vi "Average_IBP_curves_baseline.vi"(0 "I in":dbl[](array[numeric]), 1 "Averaged P(B) In":dbl[][](array[numeric]), 2 "Counter":i8, 3 "B0":dbl, 5 "Averaged I(B) In":dbl[][](array[numeric]), 7 "t in":dbl[](array[numeric]), 9 "B in":dbl[](array[numeric]), 11 "Averaged dt in":dbl[][](array[numeric]), 12 "Up/Down":bool, 13 "Sample area(mm^2)":dbl, 14 "B array":dbl[](array[numeric])) -> (4 "Averaged I(B) out":dbl[][](array[numeric]), 6 "Averaged dt Out":dbl[][](array[numeric]), 8 "Averaged P(B) Out":dbl[][](array[numeric]), 10 "BaselineSubtracted I(B)":dbl[][](array[numeric]))   [LabVIEW 2015]
uses:
  <vilib>/Analysis/baseanly.llb/Mean (DBL).vi
  <vilib>/Analysis/NI_AALBase.lvlib
  <vilib>/gmath/NI_Gmath.lvlib
panel:
  out "yi":dbl[](array[numeric]) format="%_6g"
  out "Down":cluster{"B array":dbl[], dbl[]}(graph)
  out "XY Graph 2":cluster{"B in":dbl[], "I in":dbl[]}(graph)
  out "Up":cluster{"B array":dbl[], dbl[]}(graph)
  out "subarray 2":dbl[](array[numeric])
  out "subarray":dbl[](array[numeric])
  out "Sorted array":dbl[][](array[numeric]) format="%.5f"
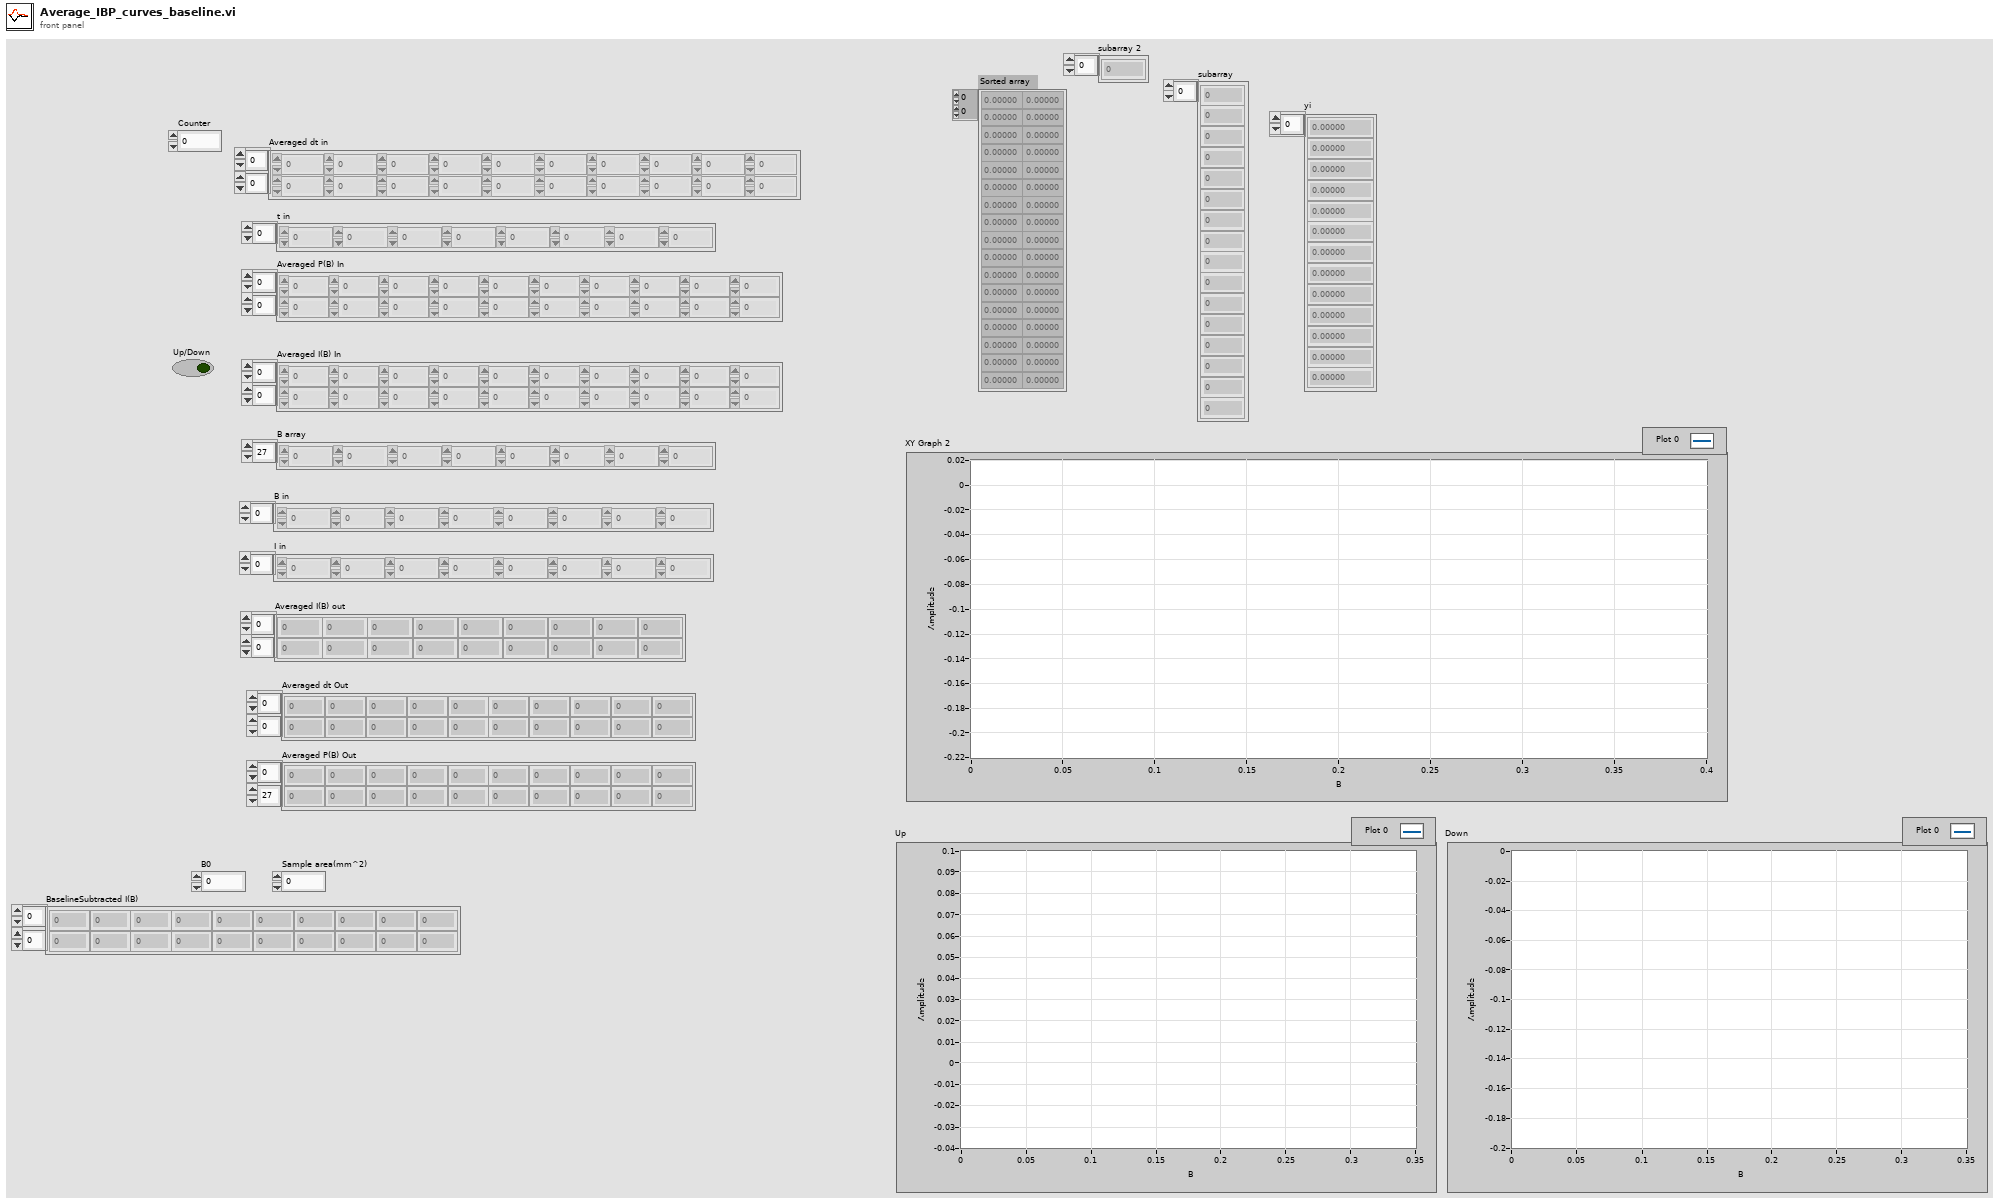
[diagram p1: front panel]
types:
  T1 = cluster{"B array":dbl[], "BaselineSubtracted I(B)":dbl[]}
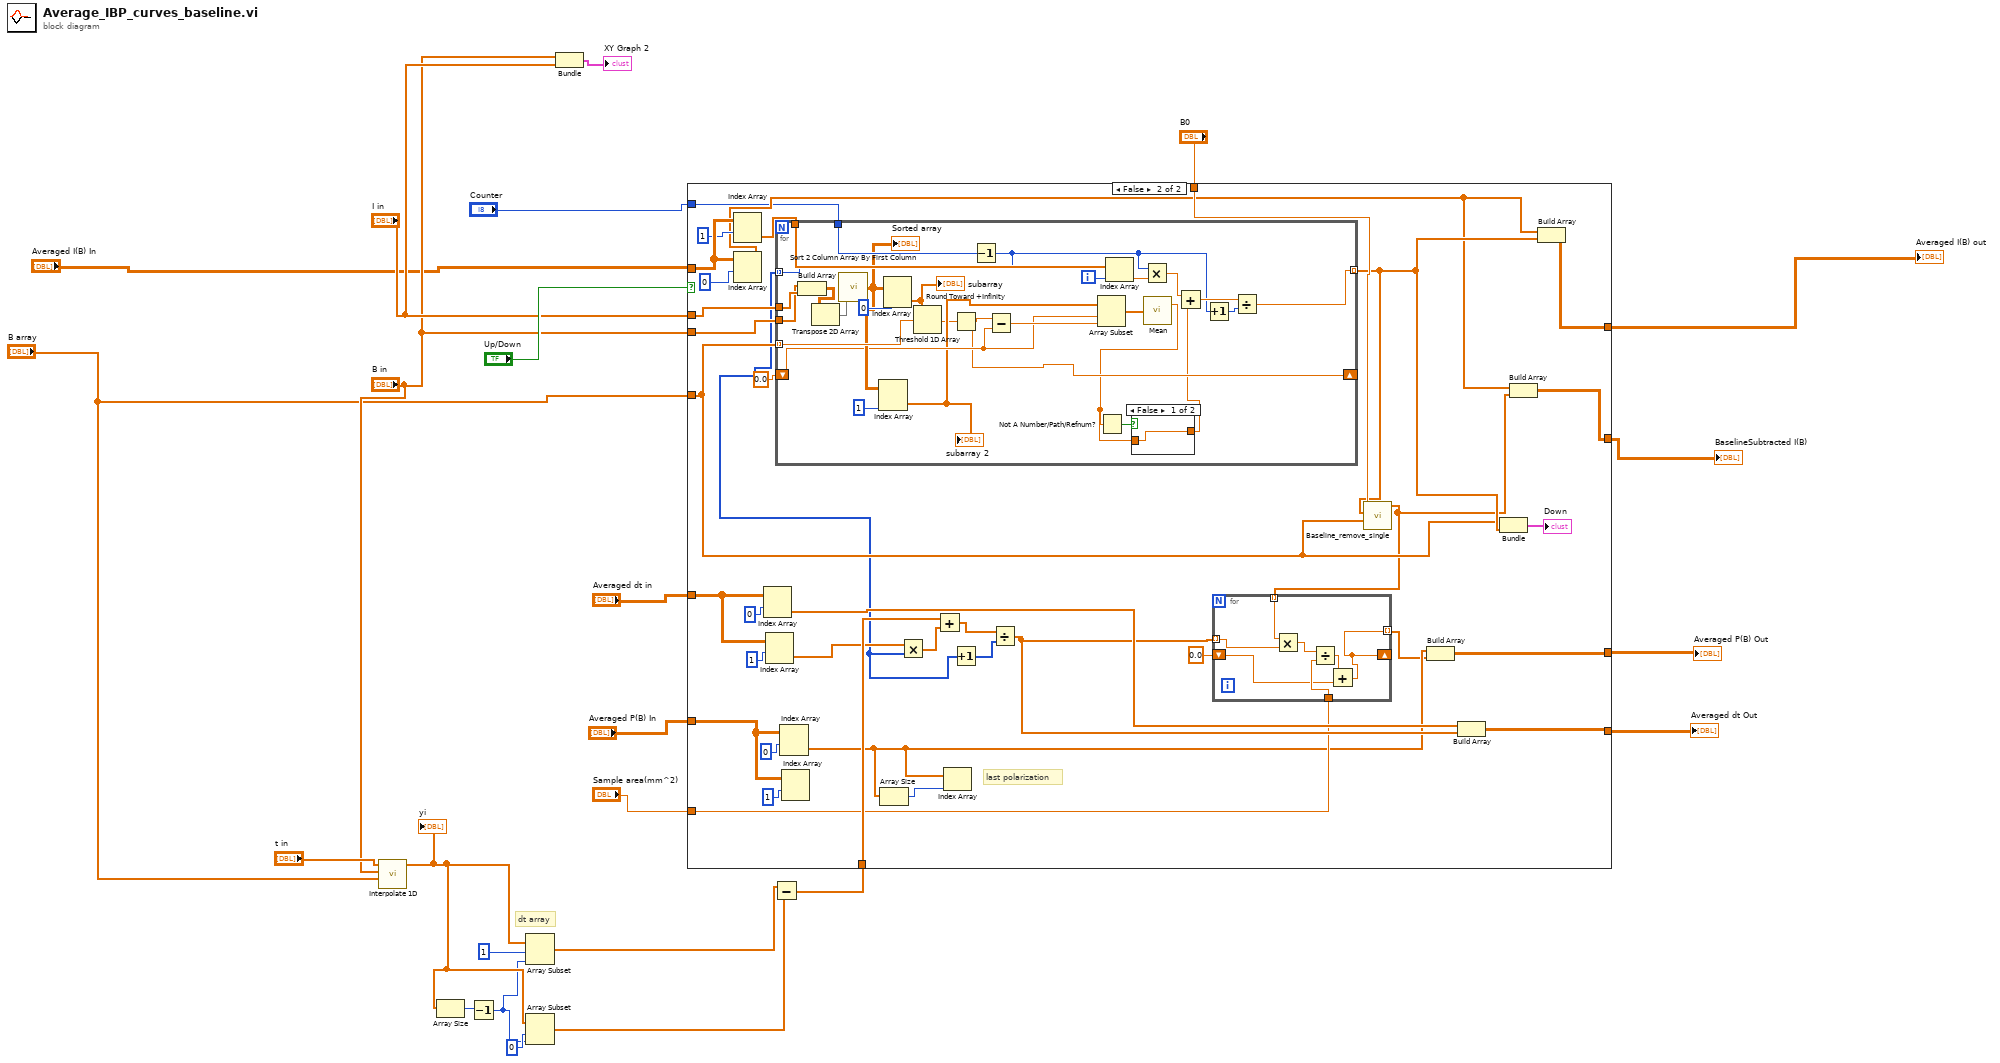
[diagram p0: block diagram]
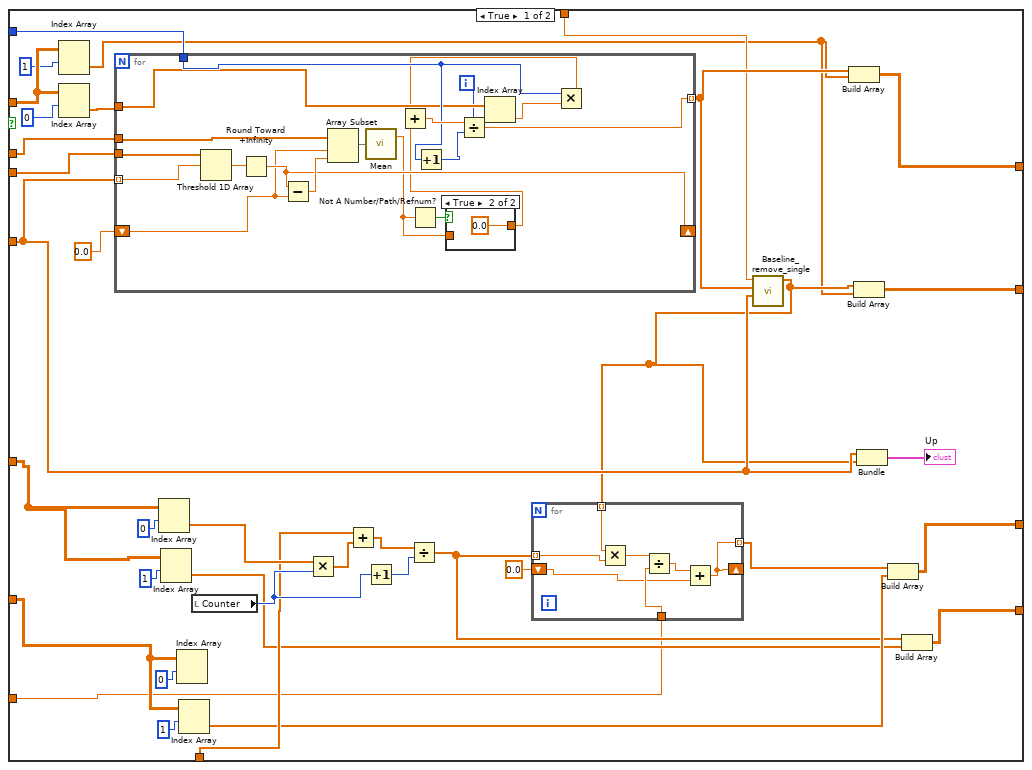
[diagram p2: hidden frame]
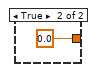
[diagram p4: hidden frame]
diagram:
  # "dt array"
  n1 = call <vilib>:"Interpolate 1D.vi"("xi"="B array", "X"="B in", "Y"="t in") -> ("yi"=w9:dbl[])  [unwired: 6 in, 2 out]
  "yi" <- w9
  n2 = Array Size(array=w9) -> (size(s)=w12:i32)
  n3 = Decrement(x=w12) -> (x-1=w5:i32)
  n4 = Array Subset(array=w9, index=1, length=w5) -> (w8:dbl[])
  n5 = Array Subset(array=w9, index=0, length=w5) -> (w7:dbl[])
  n6 = Bundle("B in"="B in", "I in"="I in") -> (→"XY Graph 2":cluster{"B in":dbl[], "I in":dbl[]})  [unwired: 1 in]
  n7 = Subtract(x=w8, y=w7) -> (x-y=w15:dbl[])
  n8 = case shown="False" "Up/Down" {
    tunnel: "Averaged I(B) In" -> [w56 w123]
    tunnel: "I in" -> [w58 w124]
    tunnel: "B in" -> [w39 w108]
    tunnel: "Counter" -> [w57 w90]
    tunnel: "B array" -> [w28 w94]
    tunnel: [w55 w97] -> w24
    tunnel: "Averaged dt in" -> [w46 w115]
    tunnel: "Averaged P(B) In" -> [w45 w114]
    tunnel: w15 -> [w44 w113]
    tunnel: [w42 w112] -> w19
    tunnel: [w40 w109] -> w18
    tunnel: "Sample area(mm^2)" -> [w31 w102]
    tunnel: "B0" -> [w29 w96]
    tunnel: [w25 w91] -> w1
    frame True {
      n9 = Index Array(array=w56, index (row)=1 ("disabled index (col)")) -> (element=w26:dbl[])  [unwired: 1 in]
      n10 = Index Array(array=w56, index (row)=0 ("disabled index (col)")) -> (element=w60:dbl[])  [unwired: 1 in]
      n11 = for {
        tunnel: w60 -> [w79]
        tunnel: w28 -> [w69] mode=indexing
        tunnel: w39 -> [w86]
        shift-right: [w74] -> _
        shift-left: 0.0 -> [w73]
        tunnel: w58 -> [w85]
        tunnel: w57 -> [w81]
        tunnel: [w80] -> w30 mode=indexing
        i -> [w78]
        n12 = Threshold 1D Array(2:w69, 3:w86) -> (0:w75:dbl)  [unwired: 1 in]
        n13 = Round Toward +Infinity(x=w75) -> (ceil(x): smallest int >= x=w74:dbl)
        n14 = Subtract(x=w74, y=w73) -> (x-y=w84:dbl)
        n15 = Array Subset(array=w85, index=w73, length=w84) -> (w76:dbl[])
        n16 = call-poly <vilib>:"Mean.vi"("X"=w76) -> ("mean"=w71:dbl)  [unwired: 1 out]
        n17 = Not A Number/Path/Refnum?(number/path/refnum=w71) -> (NaN/Path/Refnum?=w72:bool)
        n18 = Increment(x=w81) -> (x+1=w82:i8)
        n19 = case shown="True" w72 {
          tunnel: [w87 0.0] -> w70
          tunnel: w71 -> [w87 _]
          frame False {
          }
          frame True {
          }
        }
        n20 = Index Array(array=w79, index=w78) -> (element=w77:dbl)
        n21 = Multiply(x=w81, y=w77) -> (x*y=w68:dbl)
        n22 = Add(x=w68, y=w70) -> (x+y=w83:dbl)
        n23 = Divide(x=w83, y=w82) -> (x/y=w80:dbl)
      }
      n24 = Index Array(array=w46, index (row)=0 ("disabled index (col)")) -> (element=w47:dbl[])  [unwired: 1 in]
      n25 = Index Array(array=w46, index (row)=1 ("disabled index (col)")) -> (element=w41:dbl[])  [unwired: 1 in]
      n26 = Index Array(array=w45, index (row)=0 ("disabled index (col)")) -> ()  [unwired: 1 in, 1 out]
      n27 = Index Array(array=w45, index (row)=1 ("disabled index (col)")) -> (element=w43:dbl[])  [unwired: 1 in]
      n28 = local read "Counter"() -> (w49:i8)
      n29 = Multiply(x=w47, y=w49) -> (x*y=w48:dbl[])
      n30 = Add(x=w44, y=w48) -> (x+y=w50:dbl[])
      n31 = Increment(x=w49) -> (x+1=w51:i8)
      n32 = Divide(x=w50, y=w51) -> (x/y=w34:dbl[])
      n33 = call "Baseline_remove_single.vi"("B array"=w28, "I(B) in"=w30, "B0"=w29) -> ("BaselineSubtracted I(B)"=w27:dbl[])  [unwired: 7 in, 1 out]
      n34 = for {
        shift-right: [w62] -> _
        shift-left: 0.0 -> [w61]
        tunnel: [w62] -> w32 mode=indexing
        tunnel: w27 -> [w67] mode=indexing
        tunnel: w34 -> [w66] mode=indexing
        tunnel: w31 -> [w65]
        n35 = Multiply(x=w67, y=w66) -> (x*y=w64:dbl)
        n36 = Divide(x=w64, y=w65) -> (x/y=w63:dbl)
        n37 = Add(x=w63, y=w61) -> (x+y=w62:dbl)
      }
      n38 = Build Array(w30, w26) -> (w55:dbl[][])
      n39 = Build Array(w27, w26) -> (w25:dbl[][])
      n40 = Bundle("B array"=w28, "BaselineSubtracted I(B)"=w27) -> (→"Up":T1)  [unwired: 1 in]
      n41 = Build Array(w32, w43) -> (w42:dbl[][])
      n42 = Build Array(w34, w41) -> (w40:dbl[][])
    }
    frame False {
      # "last polarization"
      n43 = Index Array(array=w123, index (row)=1 ("disabled index (col)")) -> (element=w122:dbl[])  [unwired: 1 in]
      n44 = Index Array(array=w123, index (row)=0 ("disabled index (col)")) -> (element=w92:dbl[])  [unwired: 1 in]
      n45 = Index Array(array=w115, index (row)=0 ("disabled index (col)")) -> (element=w110:dbl[])  [unwired: 1 in]
      n46 = Index Array(array=w115, index (row)=1 ("disabled index (col)")) -> (element=w111:dbl[])  [unwired: 1 in]
      n47 = for {
        tunnel: w122 -> [w153]
        tunnel: w94 -> [w159] mode=indexing
        tunnel: w108 -> [w148]
        shift-right: [w138] -> _
        shift-left: 0.0 -> [w141]
        tunnel: w124 -> [w149]
        tunnel: w90 -> [w154]
        tunnel: [w134] -> w95 mode=indexing
        tunnel: [w133] -> w89 mode=indexing
        i -> [w152]
        n48 = Build Array(w148, w149) -> (w143:dbl[][])
        n49 = Transpose 2D Array(2D array=w143) -> (transposed array=w142:dbl[][])
        n50 = call "Sort 2 Column Array By First Column.vi"("2D array to sort"=w142) -> ("Sorted array"=w145:dbl[][])
        "Sorted array" <- w145
        n51 = Index Array(array=w145, index (col)=1 ("disabled index (col)")) -> (element=w140:dbl[])  [unwired: 1 in]
        "subarray 2" <- w140
        n52 = Index Array(array=w145, index (col)=0 ("disabled index (col)")) -> (element=w147:dbl[])  [unwired: 1 in]
        "subarray" <- w147
        n53 = Threshold 1D Array(2:w159, 3:w147) -> (0:w139:dbl)  [unwired: 1 in]
        n54 = Round Toward +Infinity(x=w139) -> (ceil(x): smallest int >= x=w138:dbl)
        n55 = Decrement(x=w154) -> (x-1=w133:i8)
        n56 = Subtract(x=w138, y=w141) -> (x-y=w158:dbl)
        n57 = Array Subset(array=w140, index=w141, length=w158) -> (w150:dbl[])
        n58 = Index Array(array=w153, index=w152) -> (element=w151:dbl)
        n59 = Multiply(x=w133, y=w151) -> (x*y=w157:dbl)
        n60 = call-poly <vilib>:"Mean.vi"("X"=w150) -> ("mean"=w136:dbl)  [unwired: 1 out]
        n61 = Not A Number/Path/Refnum?(number/path/refnum=w136) -> (NaN/Path/Refnum?=w137:bool)
        n62 = case shown="False" w137 {
          tunnel: [w160 0.0] -> w135
          tunnel: w136 -> [w160 _]
          frame False {
          }
          frame True {
          }
        }
        n63 = Add(x=w157, y=w135) -> (x+y=w156:dbl)
        n64 = Increment(x=w133) -> (x+1=w155:i8)
        n65 = Divide(x=w156, y=w155) -> (x/y=w134:dbl)
      }
      n66 = Index Array(array=w114, index (row)=0 ("disabled index (col)")) -> (element=w101:dbl[])  [unwired: 1 in]
      n67 = Index Array(array=w114, index (row)=1 ("disabled index (col)")) -> ()  [unwired: 1 in, 1 out]
      n68 = Array Size(array=w101) -> (size(s)=w100:i32)
      n69 = Multiply(x=w111, y=w89) -> (x*y=w116:dbl[])
      n70 = Add(x=w113, y=w116) -> (x+y=w117:dbl[])
      n71 = Index Array(array=w101, index=w100) -> ()  [unwired: 1 out]
      n72 = Increment(x=w89) -> (x+1=w118:i8[])
      n73 = Divide(x=w117, y=w118) -> (x/y=w103:dbl[])
      n74 = call "Baseline_remove_single.vi"("B array"=w94, "I(B) in"=w95, "B0"=w96) -> ("BaselineSubtracted I(B)"=w93:dbl[])  [unwired: 7 in, 1 out]
      n75 = for {
        tunnel: w103 -> [w131] mode=indexing
        tunnel: w93 -> [w130] mode=indexing
        shift-right: [w128] -> _
        shift-left: 0.0 -> [w126]
        tunnel: [w128] -> w98 mode=indexing
        tunnel: w102 -> [w127]
        n76 = Multiply(x=w130, y=w131) -> (x*y=w132:dbl)
        n77 = Divide(x=w132, y=w127) -> (x/y=w129:dbl)
        n78 = Add(x=w129, y=w126) -> (x+y=w128:dbl)
      }
      n79 = Build Array(w101, w98) -> (w112:dbl[][])
      n80 = Build Array(w110, w103) -> (w109:dbl[][])
      n81 = Bundle("B array"=w94, w95) -> (→"Down":cluster{"B array":dbl[], dbl[]})  [unwired: 1 in]
      n82 = Build Array(w92, w93) -> (w91:dbl[][])
      n83 = Build Array(w92, w95) -> (w97:dbl[][])
    }
  }
  "Averaged I(B) out" <- w24
  "Averaged P(B) Out" <- w19
  "Averaged dt Out" <- w18
  "BaselineSubtracted I(B)" <- w1
